vi "Write CellData.vi"(8 "error in":errorcluster, 10 "CellData":refnum<class "CRDS Cell Data.lvclass">[](array[class]), 11 "CRDS Data in":refnum<class "CRDS Data.lvclass">) -> (0 "error out":errorcluster, 3 "CRDS Data out":refnum<class "CRDS Data.lvclass">)   [LabVIEW 2015, in "CRDS Data.lvclass"]
uses:
  CRDS Data.lvclass
  Cell/CRDS Cell Data.lvclass
  CRDS Data.lvclass/CRDS Data.ctl
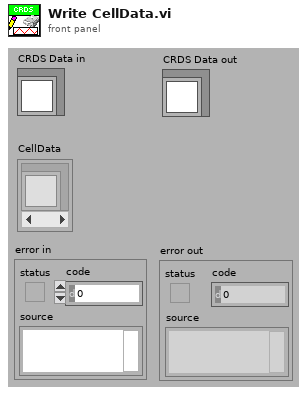
[diagram p1: front panel]
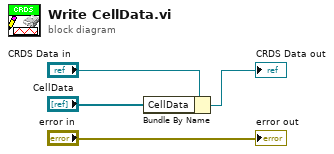
[diagram p0: block diagram]
diagram:
  n1 = Bundle By Name(cluster="CRDS Data in", "CellData"="CellData") -> (→"CRDS Data out":refnum<class "CRDS Data.lvclass">)
  "error out" <- "error in"
